vi "Add VI to Tab Control.vi"(8 "error in (no error)":errorcluster, 9 "VI Refnum":refnum<vi>, 11 "TabControl in":refnum<vi>) -> (0 "error out":errorcluster)   [LabVIEW 2020, in "RxnRover.lvlib"]
doc: "Adds the VI to the first visible page of the tab control given, assuming the first control on the page is a subpanel."
uses:
  RxnRover.lvlib
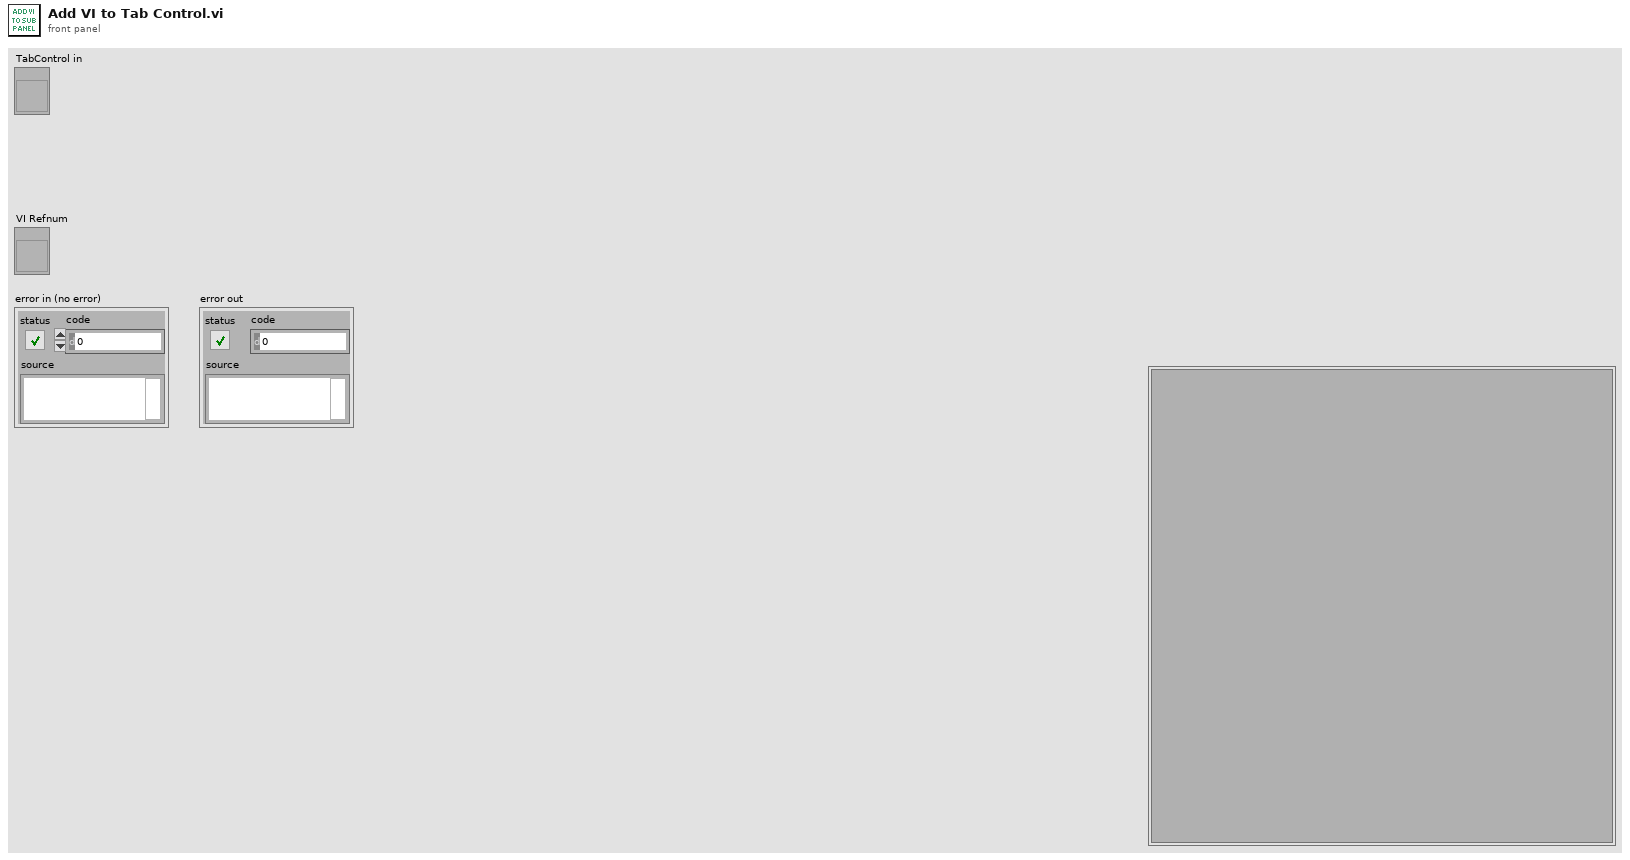
[diagram p1: front panel]
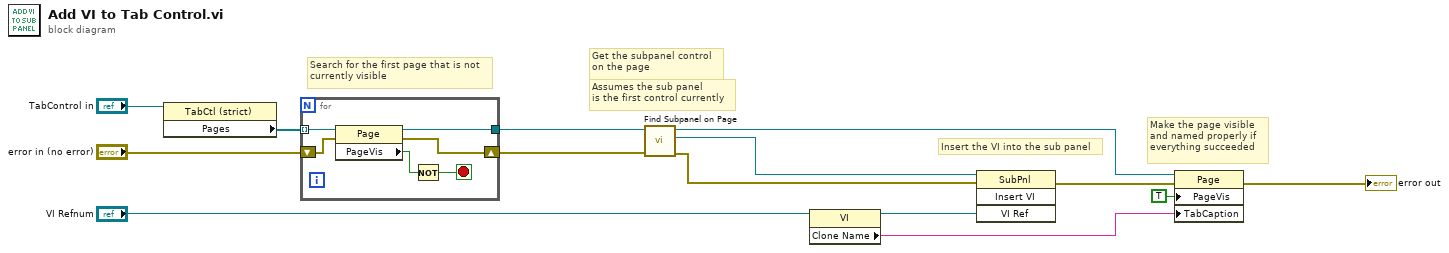
[diagram p0: block diagram]
diagram:
  # "Assumes the sub panel\nis the first control currently"
  # "Get the subpanel control\non the page"
  # "Make the page visible \nand named properly if\neverything succeeded"
  # "Insert the VI into the sub panel"
  # "Search for the first page that is not\ncurrently visible"
  n1 = property on="Property Node" class="TabCtl (strict)"(reference="TabControl in") -> ("Pages"=w10:refnum<vi>[])  [unwired: 1 in, 2 out]
  n2 = for {
    shift-right: [w18] -> w11
    shift-left: "error in (no error)" -> [w19]
    tunnel: w10 -> [w20] mode=indexing
    tunnel: [w17] -> w12
    stop <- w15 stop-if-true
    n3 = property class="Page"(reference=w20, error in=w19) -> (reference out=w17:refnum<vi>, error out=w18:errorcluster, "PageVis"=w16:bool)
    n4 = Not(x=w16) -> (.not. x?=w15:bool)
  }
  n5 = call "Find Subpanel on Page.vi"("error in (no error)"=w11, "Page in"=w12) -> ("error out"=w1:errorcluster, "Sub panel reference"=w2:refnum<vi>, "Page out"=w6:refnum<vi>)  [unwired: 7 in]
  n6 = property class="VI"(reference="VI Refnum") -> (reference out=w4:refnum<vi>, "Clone Name"=w3:string)  [unwired: 1 in, 1 out]
  n7 = invoke class="SubPnl" method="Insert VI"(reference=w2, error in=w1, "VI Ref"=w4) -> (error out=w14:errorcluster)  [unwired: 1 in, 3 out]
  n8 = property class="Page"(reference=w6, error in=w14, "PageVis"=TRUE ("Page Visible"), "TabCaption"=w3) -> (error out=→"error out":errorcluster)  [unwired: 1 out]
